vi "多幅图像写入AVI.vi"() -> ()   [LabVIEW 2018]
uses:
  <vilib>/vision/NI_Vision_Development_Module.lvlib
panel:
  out "error out":errorcluster
  in  "错误输入":errorcluster
  in  "路径":path
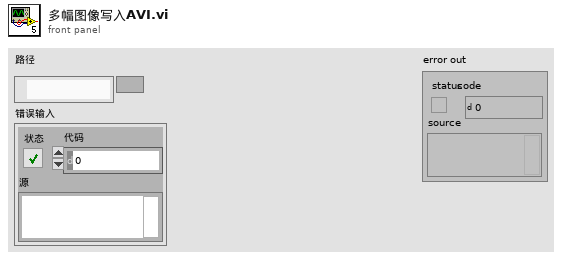
[diagram p1: front panel]
types:
  T1 = typedef "Image Type" = u32
  T2 = typedef "IMAQ Image.ctl" = refnum<image>
  T3 = typedef "IMAQ AVI2 Refnum.ctl" = refnum<k20>
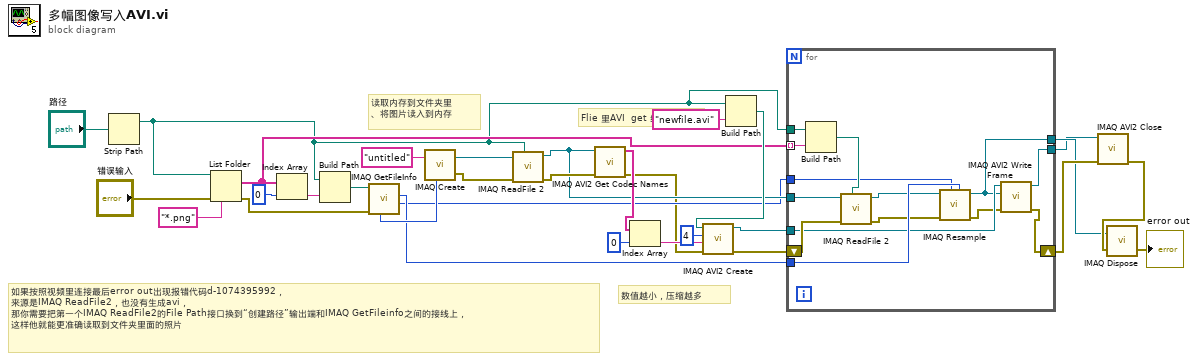
[diagram p0: block diagram]
diagram:
  # "如果按照视频里连接最后error out出现报错代码d-1074395992，\n来源是IMAQ ReadFile2，也没有生成avi，\n那你需要把第一个IMAQ ReadFile2的File Path接口换到“创建路径”输出端和IMAQ GetFileinfo之间的接线上，\n这样他就能更准确读取到文件夹里面的照片"
  # "数值越小，压缩越多"
  # "Flie 里AVI  get 编码器"
  # "读取内存到文件夹里\n、将图片读入到内存"
  n1 = Strip Path(path="路径") -> (stripped path=w1:path)  [unwired: 1 out]
  n2 = List Folder(path=w1, pattern="*.png" ("类型"), error in="错误输入") -> (filenames=w13:string[], error out=w24:errorcluster)  [unwired: 1 in, 2 out]
  n3 = Index Array(array=w13, index=0 ("索引")) -> (element=w28:string)
  n4 = Build Path(base path=w1, name or relative path=w28) -> (appended path=w2:path)
  n5 = call "IMAQ GetFileInfo"("error in (no error)"=w24, "File Path"=w2) -> ("Y Resolution"=w10:i32, "X Resolution"=w11:i32, "Image Type"=w25:T1)  [unwired: 3 in, 4 out]
  n6 = call "IMAQ Create"("Image Name"="untitled", "Image Type"=w25) -> ("New Image"=w23:T2, "error out"=w22:errorcluster)  [unwired: 3 in]
  n7 = call "IMAQ ReadFile 2"("File Path"=w1, "error in (no error)"=w22, "Image"=w23) -> ("error out"=w21:errorcluster, "Image Out"=w14:T2)  [unwired: 4 in, 3 out]
  n8 = call "IMAQ AVI2 Get Codec Names"("error in (no error)"=w21, "Image"=w14) -> ("error out"=w4:errorcluster, "Codec Names"=w20:string[])  [unwired: 8 in]
  n9 = Index Array(array=w20, index=0 ("索引")) -> (element=w18:string)
  n10 = Build Path(base path=w1, name or relative path="newfile.avi" ("名称或相对路径")) -> (appended path=w16:path)
  n11 = call "IMAQ AVI2 Create"("error in (no error)"=w4, "Codec"=w18, "Frames Per Second"=u32 4, "AVI Path"=w16) -> ("error out"=w12:errorcluster, "AVI Refnum"=w9:T3)  [unwired: 6 in]
  n12 = for {
    tunnel: w1 -> [w45]
    tunnel: w14 -> [w44]
    tunnel: w13 -> [w42] mode=indexing
    shift-right: [w34] -> w8
    shift-left: w12 -> [w41]
    tunnel: w11 -> [w40]
    tunnel: w10 -> [w39]
    tunnel: w9 -> [w37]
    tunnel: [w33] -> w6
    tunnel: [w32] -> w3
    n13 = Build Path(base path=w45, name or relative path=w42) -> (appended path=w43:path)
    n14 = call "IMAQ ReadFile 2"("File Path"=w43, "error in (no error)"=w41, "Image"=w44) -> ("error out"=w38:errorcluster, "Image Out"=w36:T2)  [unwired: 4 in, 3 out]
    n15 = call "IMAQ Resample"("X Resolution"=w40, "Y Resolution"=w39, "error in (no error)"=w38, "Image Src"=w36) -> ("error out"=w35:errorcluster, "Image Dst Out"=w33:T2)  [unwired: 6 in]
    n16 = call "IMAQ AVI2 Write Frame"("error in (no error)"=w35, "Image"=w33, "AVI Refnum"=w37) -> ("error out"=w34:errorcluster, "AVI Refnum (duplicate)"=w32:T3)  [unwired: 6 in, 1 out]
  }
  n17 = call "IMAQ AVI2 Close"("error in (no error)"=w8, "AVI Refnum"=w3) -> ("error out"=w7:errorcluster)  [unwired: 9 in]
  n18 = call "IMAQ Dispose"("Image"=w6, "error in (no error)"=w7) -> ("error out"=→"error out":errorcluster)  [unwired: 4 in]
